vi "Crea curva rendimento.vi"() -> (0 "Strings []":string[](array[string]), 1 "Text.Text":string, 2 "Array":dbl[][](array[numeric]), 3 "XY Graph":cluster{"X":dbl[], "Y":dbl[]}[](graph))   [LabVIEW 2019]
uses:
  <vilib>/Utility/file.llb/Read Delimited Spreadsheet (string).vi
  <vilib>/Utility/file.llb/Write Delimited Spreadsheet (DBL).vi
  <vilib>/Analysis/NI_AALPro.lvlib
  <vilib>/gmath/NI_Gmath.lvlib
panel:
  in  "LISTA CURVE ESISTENTI":string(combo)
  out "Array 2":dbl[][](array[numeric])
  in  "Open Button":bool
  out "cover":bool
  in  "exit":bool
  in  "Save Button":bool
  in  "P1[kW]":dbl[](array[numeric]) format="%0.2f"
  in  "Rend %":dbl[](array[numeric]) format="%0.2f"
  # "CURVA P1 - RENDIMENTO"
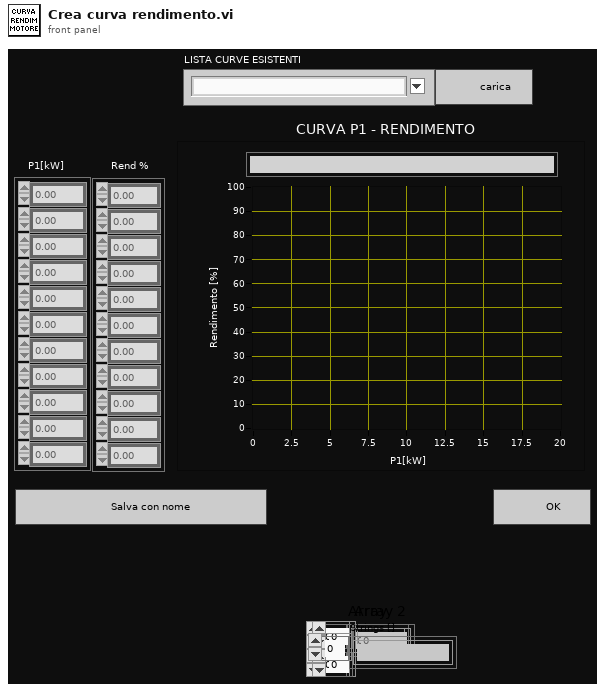
[diagram p1: front panel]
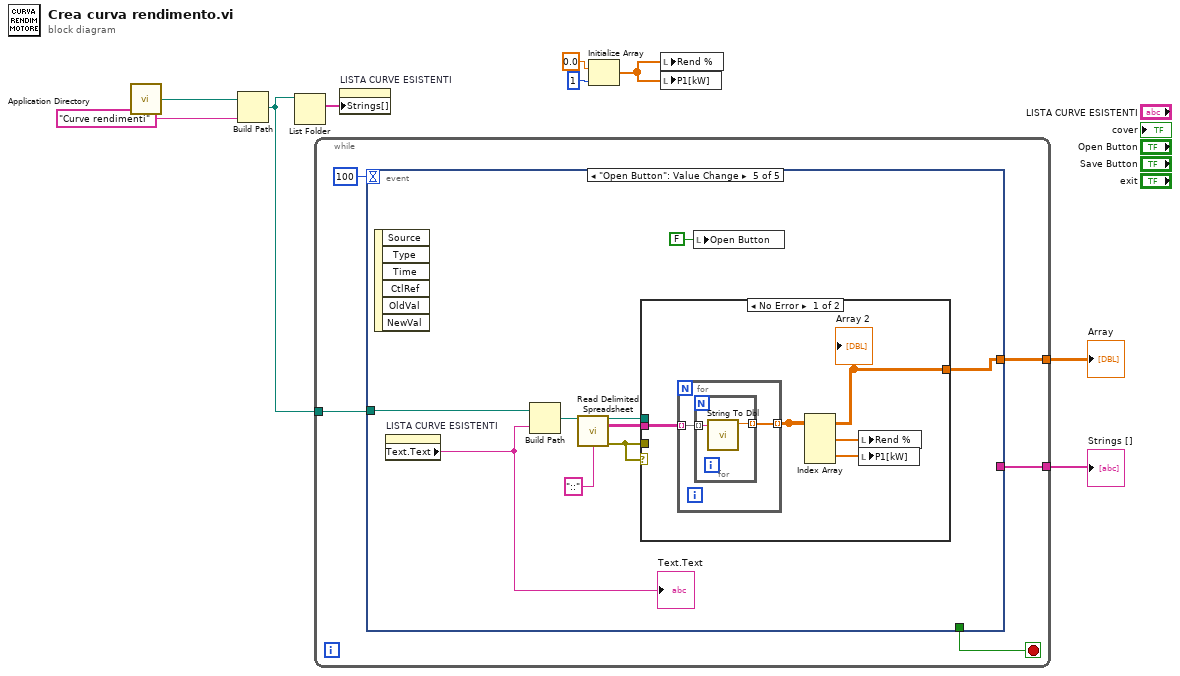
[diagram p0: block diagram]
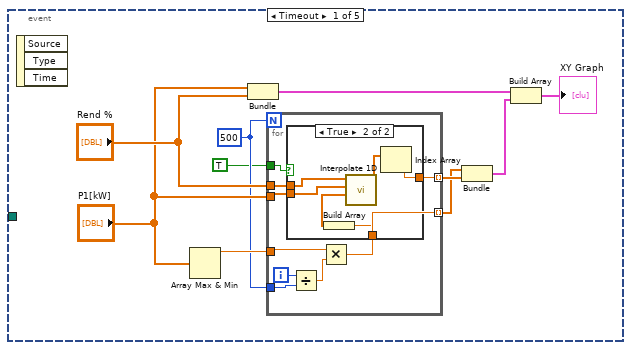
[diagram p2: hidden frame]
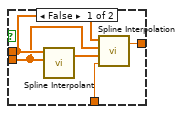
[diagram p3: hidden frame]
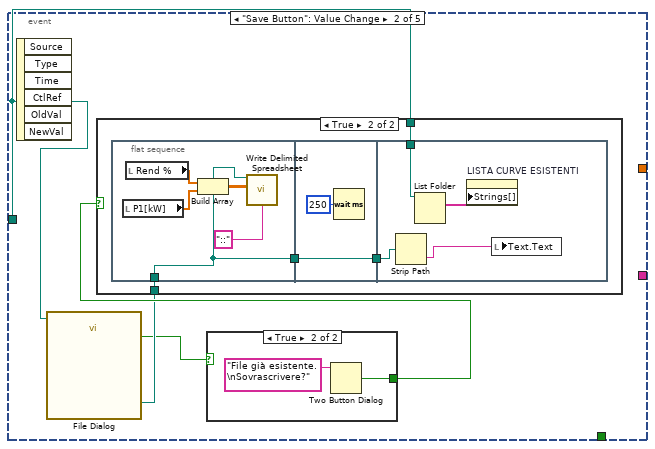
[diagram p4: hidden frame]
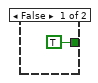
[diagram p6: hidden frame]
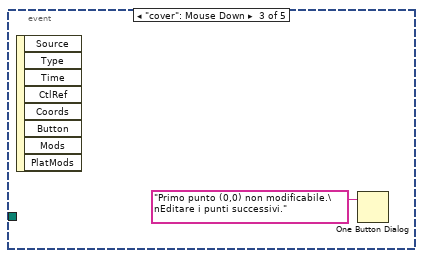
[diagram p7: hidden frame]
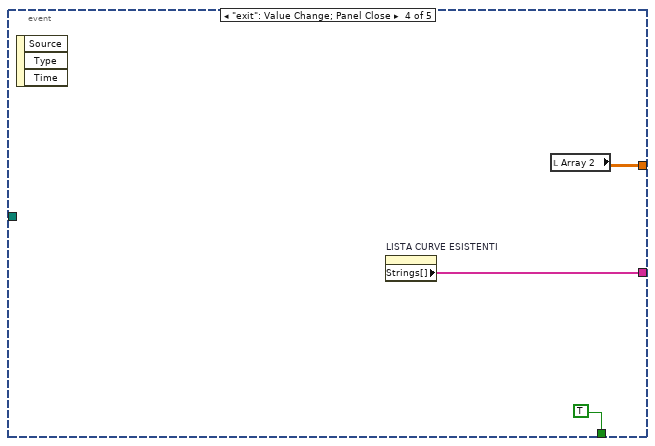
[diagram p8: hidden frame]
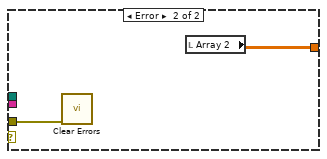
[diagram p9: hidden frame]
diagram:
  n1 = call <vilib>:"Application Directory.vi"() -> ("Application Directory"=w5:path)
  n2 = Build Path(base path=w5, name or relative path="Curve rendimenti") -> (appended path=w2:path)
  n3 = List Folder(path=w2) -> (filenames=w3:string[])  [unwired: 3 in, 3 out]
  n4 = while {
    tunnel: [w12] -> w6
    tunnel: w2 -> [w11]
    tunnel: [w10] -> w1
    stop <- w13 stop-if-true
    n5 = event shown="[4] \"Open Button\": Value Change" {
      selector: _ -> [_ _ _ _ _]
      dyn-events: _ -> [_ _ _ _ _]
      timeout: 100 -> [_ _ _ _ _]
      tunnel: [_ _ _ TRUE _] -> w13
      tunnel: [_ _ _ w69 w76] -> w12
      tunnel: w11 -> [_ w47 _ _ w74]
      tunnel: [_ _ _ w68 _] -> w10
      event Timeout {
        w21 = 500
        n6 = event-data() -> ()  [unwired: 1 in, 3 out]
        n7 = Array Max & Min(array="P1[kW]") -> (max value=w23:dbl)  [unwired: 3 out]
        n8 = Bundle("P1[kW]"="P1[kW]", "Rend %"="Rend %") -> (w18:cluster{"P1[kW]":dbl[], "Rend %":dbl[]})  [unwired: 1 in]
        n9 = for {
          N: w21 -> [_]
          tunnel: "P1[kW]" -> [w28]
          tunnel: "Rend %" -> [w29]
          tunnel: w23 -> [w32]
          tunnel: [w26] -> w20 mode=indexing
          tunnel: [w27] -> w19 mode=indexing
          tunnel: w21 -> [w30]
          tunnel: TRUE -> [w25]
          i -> [w33]
          n10 = Divide(x=w33, y=w30) -> (x/y=w31:dbl)
          n11 = Multiply(x=w32, y=w31) -> (x*y=w27:dbl)
          n12 = case shown="True" w25 {
            tunnel: w29 -> [w37 w44]
            tunnel: w28 -> [w36 w43]
            tunnel: w27 -> [w35 w42]
            tunnel: [w34 w39] -> w26
            frame False {
              n13 = call <vilib>:"Spline Interpolant.vi"("X"=w36, "Y"=w37) -> ("Interpolant"=w38:dbl[])  [unwired: 2 in, 1 out]
              n14 = call <vilib>:"Spline Interpolation.vi"("x value"=w35, "Interpolant"=w38, "X"=w36, "Y"=w37) -> ("interpolation value"=w34:dbl)  [unwired: 1 out]
            }
            frame True {
              n15 = Build Array(w42) -> (w41:dbl[])
              n16 = call <vilib>:"Interpolate 1D.vi"("xi"=w41, "X"=w43, "Y"=w44) -> ("yi"=w40:dbl[])  [unwired: 6 in, 2 out]
              n17 = Index Array(array=w40) -> (element=w39:dbl)  [unwired: 1 in]
            }
          }
        }
        n18 = Bundle(w19, w20) -> (w16:cluster{dbl[], dbl[]})  [unwired: 1 in]
        n19 = Build Array(w18, w16) -> (→"XY Graph":cluster{"P1[kW]":dbl[], "Rend %":dbl[]}[])
      }
      event "Save Button": Value Change {
        n20 = event-data() -> ()  [unwired: 1 in, 6 out]
        n21 = call "File Dialog"("start path"=w47) -> ("selected path"=w46:path, "exists"=w45:bool)  [unwired: 11 in, 2 out]
        n22 = case shown="True" w45 {
          tunnel: [TRUE ("T button?") w66] -> w48
          frame False {
          }
          frame True {
            n23 = Two Button Dialog(message="File già esistente.\nSovrascrivere?") -> (T button?=w66:bool)  [unwired: 2 in]
          }
        }
        n24 = case shown="True" w48 {
          tunnel: w47 -> [_ w52]
          tunnel: w46 -> [_ w51]
          frame False {
          }
          frame True {
            n25 = flat-sequence {
              tunnel: w51 -> [w53]
              tunnel: [w53] -> w50
              tunnel: w50 -> [w58]
              tunnel: [w58] -> w49
              tunnel: w52 -> [w62]
              tunnel: w49 -> [w61]
              frame #0 {
                n26 = local read "P1[kW]"() -> (w56:dbl[])
                n27 = local read "Rend %"() -> (w57:dbl[])
                n28 = Build Array(w57, w56) -> (w55:dbl[][])
                n29 = call-poly <vilib>:"Write Delimited Spreadsheet.vi"("file path (dialog if empty)"=w53, "2D data"=w55, "delimiter (\\t)"="::" ("delimiter (\\t)")) -> ()  [unwired: 11 in, 2 out]
              }
              frame #1 {
                n30 = Wait (ms)(milliseconds to wait=u32 250) -> ()  [unwired: 1 out]
              }
              frame #2 {
                n31 = Strip Path(path=w61) -> (name=w60:string)  [unwired: 1 out]
                n32 = List Folder(path=w62) -> (filenames=w63:string[])  [unwired: 3 in, 3 out]
                n33 = property on="LISTA CURVE ESISTENTI" class="CmbBox"("Strings[]"=w63) -> ()  [unwired: 2 in, 2 out]
                n34 = local write "Text.Text"(w60) -> ()
              }
            }
          }
        }
      }
      event "cover": Mouse Down {
        n35 = event-data() -> ()  [unwired: 1 in, 8 out]
        n36 = One Button Dialog(message="Primo punto (0,0) non modificabile.\nEditare i punti successivi.") -> ()  [unwired: 1 in, 1 out]
      }
      event "exit": Value Change; Panel Close {
        n37 = event-data() -> ()  [unwired: 1 in, 3 out]
        n38 = property on="LISTA CURVE ESISTENTI" class="CmbBox"() -> ("Strings[]"=w68:string[])  [unwired: 2 in, 2 out]
        n39 = local read "Array 2"() -> (w69:dbl[][])
      }
      event "Open Button": Value Change {
        n40 = event-data() -> ()  [unwired: 1 in, 6 out]
        n41 = property on="LISTA CURVE ESISTENTI" class="CmbBox"() -> ("Text.Text"=w73:string)  [unwired: 2 in, 2 out]
        "Text.Text" <- w73
        n42 = Build Path(base path=w74, name or relative path=w73) -> (appended path=w72:path)
        n43 = call-poly <vilib>:"Read Delimited Spreadsheet.vi"("file path (dialog if empty)"=w72, "delimiter (\\t)"="::" ("delimiter (\\t)")) -> ("new file path (Not A Path if cancelled)"=w77:path, "all rows"=w78:string[][], "error out"=w75:errorcluster)  [unwired: 8 in, 3 out]
        n44 = case shown="No Error" w75 {
          tunnel: w78 -> [w83 _]
          tunnel: w77 -> [_ _]
          tunnel: [w80 w89] -> w76
          tunnel: w75 -> [_ w88]
          frame No Error {
            n45 = for {
              tunnel: w83 -> [w85] mode=indexing
              tunnel: [w84] -> w80 mode=indexing
              n46 = for {
                tunnel: w85 -> [w87] mode=indexing
                tunnel: [w86] -> w84 mode=indexing
                n47 = call "String To Dbl.vi"("String"=w87) -> ("Numeric"=w86:dbl)  [unwired: 10 in]
              }
            }
            "Array 2" <- w80
            n48 = Index Array(array=w80) -> (element #1=w82:dbl[], element #2=w81:dbl[])  [unwired: 4 in]
            n49 = local write "Rend %"(w82) -> ()
            n50 = local write "P1[kW]"(w81) -> ()
          }
          frame Error {
            n51 = call <vilib>:"Clear Errors.vi"("error in (no error)"=w88) -> ()  [unwired: 5 in, 2 out]
            n52 = local read "Array 2"() -> (w89:dbl[][])
          }
        }
        n53 = local write "Open Button"(FALSE ("Open Button")) -> ()
      }
    }
  }
  "Array" <- w6
  "Strings []" <- w1
  n54 = property on="LISTA CURVE ESISTENTI" class="CmbBox"("Strings[]"=w3) -> ()  [unwired: 2 in, 2 out]
  n55 = Initialize Array(0.0 ("element"), 1 ("dimension size")) -> (w7:dbl[])
  n56 = local write "Rend %"(w7) -> ()
  n57 = local write "P1[kW]"(w7) -> ()
